vi "SMT_Deal.vi"(5 "Operatorname":string, 6 "Computer":string, 7 "ProdOrder":string, 8 "error in (no error)":errorcluster caption="错误输入（无错误）", 9 "Type":string, 10 "LoadID":string, 11 "Traceability 引用句柄":refnum<k24>) -> (0 "error out":errorcluster caption="错误输出", 2 "SMT_DealWI":string, 3 "Traceability 引用句柄输出":refnum<k24>)   [LabVIEW 2014, in "Traceability.lvlib"]
uses:
  D:/webservice/Traceability.dll
  Traceability.dll
  Traceability.lvlib
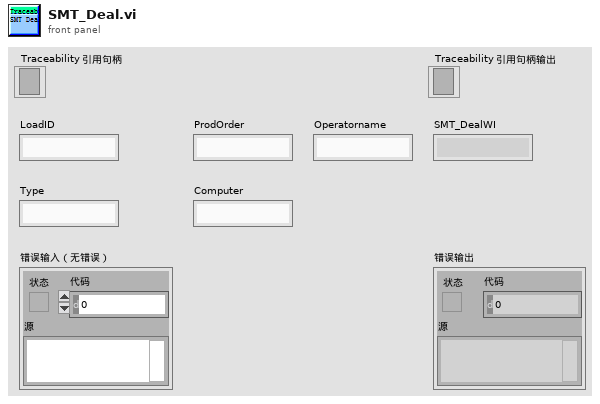
[diagram p1: front panel]
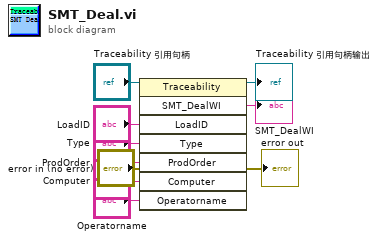
[diagram p0: block diagram]
diagram:
  n1 = invoke class="Traceability" method="SMT_DealWI"(reference="Traceability 引用句柄", error in="error in (no error)", "LoadID"="LoadID", "Type"="Type", "ProdOrder"="ProdOrder", "Computer"="Computer", "Operatorname"="Operatorname") -> (reference out=→"Traceability 引用句柄输出":refnum<k24>, error out=→"error out":errorcluster, "SMT_DealWI"=→"SMT_DealWI":string)  [unwired: 1 in, 5 out]
